vi "readTimestamp.vi"(8 "error in (no error)":errorcluster, 11 "ModbusBuffer in":refnum<class "ModbusBuffer.lvclass">) -> (0 "error out":errorcluster, 2 "Output":dbl, 3 "ModbusBuffer out":refnum<class "ModbusBuffer.lvclass">)   [LabVIEW 2016, in "RTModbus.lvlib" / "ModbusBuffer.lvclass"]
uses:
  ModbusBuffer.lvclass
  ModbusBuffer.lvclass/ModbusBuffer.ctl
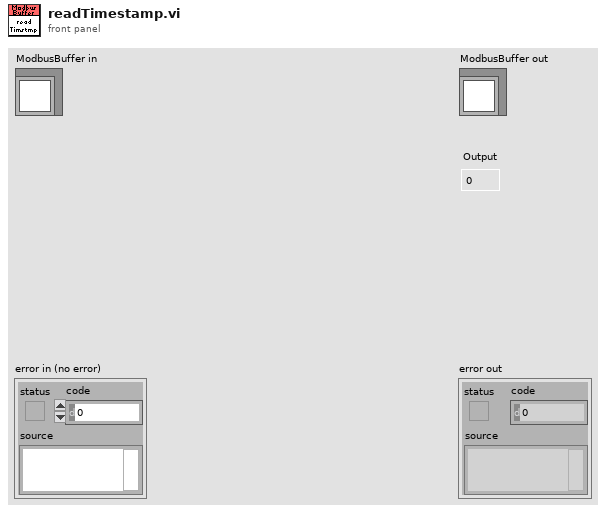
[diagram p1: front panel]
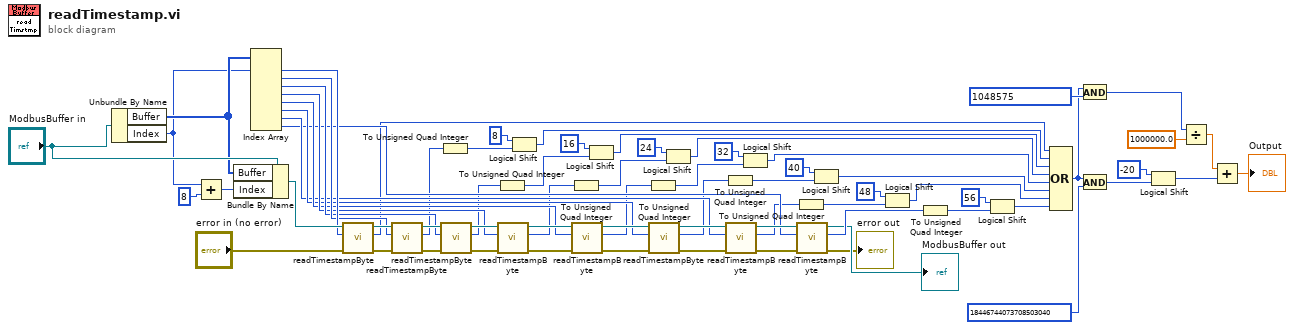
[diagram p0: block diagram]
diagram:
  n1 = Unbundle By Name("ModbusBuffer in") -> ("Buffer"=w69:u16[], "Index"=w68:i32)
  n2 = Add(x=w68, y=8) -> (x+y=w66:i32)
  n3 = Bundle By Name(cluster="ModbusBuffer in", "Buffer"=w69, "Index"=w66) -> (w44:refnum<class "ModbusBuffer.lvclass">)
  n4 = Index Array(array=w69, index #1=w68) -> (element #1=w28:u16, element #2=w27:u16, element #3=w26:u16, element #4=w25:u16, element #5=w24:u16, element #6=w23:u16, element #7=w22:u16, element #8=w21:u16)  [unwired: 7 in]
  n5 = call "readTimestampByte.vi"("error in (no error)"="error in (no error)", "Instruction"=w28, "ModbusBuffer in"=w44) -> ("error out"=w35:errorcluster, "Output"=w20:u8, "ModbusBuffer out"=w43:refnum<class "ModbusBuffer.lvclass">)  [unwired: 6 in]
  n6 = call "readTimestampByte.vi"("error in (no error)"=w35, "Instruction"=w27, "ModbusBuffer in"=w43) -> ("error out"=w34:errorcluster, "Output"=w19:u8, "ModbusBuffer out"=w42:refnum<class "ModbusBuffer.lvclass">)  [unwired: 6 in]
  n7 = To Unsigned Quad Integer(1:w19) -> (0:w59:u64)
  n8 = call "readTimestampByte.vi"("error in (no error)"=w34, "Instruction"=w26, "ModbusBuffer in"=w42) -> ("error out"=w33:errorcluster, "Output"=w18:u8, "ModbusBuffer out"=w41:refnum<class "ModbusBuffer.lvclass">)  [unwired: 6 in]
  n9 = To Unsigned Quad Integer(1:w18) -> (0:w58:u64)
  n10 = call "readTimestampByte.vi"("error in (no error)"=w33, "Instruction"=w25, "ModbusBuffer in"=w41) -> ("error out"=w32:errorcluster, "Output"=w17:u8, "ModbusBuffer out"=w40:refnum<class "ModbusBuffer.lvclass">)  [unwired: 6 in]
  n11 = Logical Shift(y=i16 8, x=w59) -> (x << y=w64:u64)
  n12 = To Unsigned Quad Integer(1:w17) -> (0:w57:u64)
  n13 = call "readTimestampByte.vi"("error in (no error)"=w32, "Instruction"=w24, "ModbusBuffer in"=w40) -> ("error out"=w31:errorcluster, "Output"=w16:u8, "ModbusBuffer out"=w39:refnum<class "ModbusBuffer.lvclass">)  [unwired: 6 in]
  n14 = Logical Shift(y=i16 16, x=w58) -> (x << y=w60:u64)
  n15 = To Unsigned Quad Integer(1:w16) -> (0:w56:u64)
  n16 = call "readTimestampByte.vi"("error in (no error)"=w31, "Instruction"=w23, "ModbusBuffer in"=w39) -> ("error out"=w30:errorcluster, "Output"=w15:u8, "ModbusBuffer out"=w38:refnum<class "ModbusBuffer.lvclass">)  [unwired: 6 in]
  n17 = Logical Shift(y=i16 24, x=w57) -> (x << y=w61:u64)
  n18 = To Unsigned Quad Integer(1:w15) -> (0:w53:u64)
  n19 = call "readTimestampByte.vi"("error in (no error)"=w30, "Instruction"=w22, "ModbusBuffer in"=w38) -> ("error out"=w29:errorcluster, "Output"=w14:u8, "ModbusBuffer out"=w37:refnum<class "ModbusBuffer.lvclass">)  [unwired: 6 in]
  n20 = Logical Shift(y=i16 32, x=w56) -> (x << y=w48:u64)
  n21 = To Unsigned Quad Integer(1:w14) -> (0:w52:u64)
  n22 = call "readTimestampByte.vi"("error in (no error)"=w29, "Instruction"=w21, "ModbusBuffer in"=w37) -> ("error out"=→"error out":errorcluster, "Output"=w13:u8, "ModbusBuffer out"=→"ModbusBuffer out":refnum<class "ModbusBuffer.lvclass">)  [unwired: 6 in]
  n23 = Logical Shift(y=i16 40, x=w53) -> (x << y=w47:u64)
  n24 = Logical Shift(y=i16 48, x=w52) -> (x << y=w46:u64)
  n25 = To Unsigned Quad Integer(1:w13) -> (0:w49:u64)
  n26 = Logical Shift(y=i16 56, x=w49) -> (x << y=w45:u64)
  n27 = Compound Arithmetic op=OR(w20, w64, w60, w61, w48, w47, w46, w45) -> (w2:u64)
  n28 = And(x=w2, y=u64 1048575) -> (x .and. y?=w8:u64)
  n29 = And(x=w2, y=u64 18446744073708503040) -> (x .and. y?=w6:u64)
  n30 = Logical Shift(y=i16 -20, x=w6) -> (x << y=w3:u64)
  n31 = Divide(x=w8, y=1000000.0) -> (x/y=w4:dbl)
  n32 = Add(x=w4, y=w3) -> (x+y=→"Output":dbl)
